vi "Query Instrument for ID and Name.vi"(0 "VISA resource name":refnum<visa-resource-name>, 11 "error in (no error)":errorcluster) -> (4 "VISA resource name out":refnum<visa-resource-name>, 6 "Logical Instrument Number":u32 max=12 step=1, 8 "Logical Instrument Name":string, 15 "error out":errorcluster)   [LabVIEW 2020, in "NH Research Regenerative Test Series.lvlib"]
doc: "Returns the <B>Logical Instrument Number</B> and <B>Logical Instrument Name</B> of the selected instrument.\n\nNOTE: The 4900 only has one logical instrument so the only valid instrument number is 1."
uses:
  NH Research Regenerative Test Series.lvlib
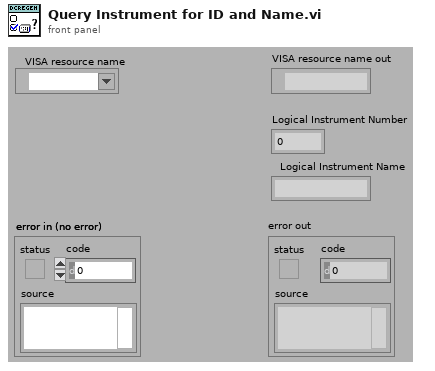
[diagram p1: front panel]
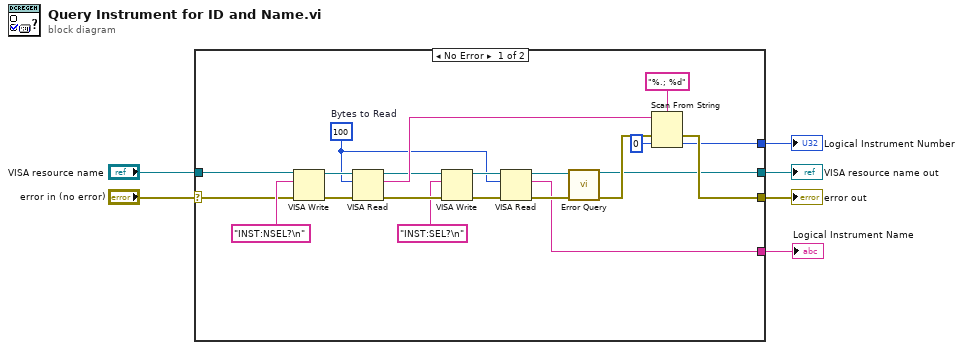
[diagram p0: block diagram]
diagram:
  n1 = case shown="No Error" "error in (no error)" {
    selector: "error in (no error)" -> [w18 w29]
    tunnel: "VISA resource name" -> [w27 w28]
    tunnel: [w20 w28] -> w5
    tunnel: [w21 w29] -> w4
    tunnel: [w7 _] -> w2
    tunnel: [w10 _] -> w1
    frame No Error {
      w9 = u32 100  # Bytes to Read
      n2 = VISA Write(VISA resource name=w27, write buffer="INST:NSEL?\n" ("Command"), error in (no error)=w18) -> (VISA resource name out=w22:refnum<visa-resource-name>, error out=w23:errorcluster)  [unwired: 1 out]
      n3 = VISA Read(VISA resource name=w22, byte count=w9, error in (no error)=w23) -> (VISA resource name out=w13:refnum<visa-resource-name>, read buffer=w26:string, error out=w15:errorcluster)  [unwired: 1 out]
      n4 = VISA Write(VISA resource name=w13, write buffer="INST:SEL?\n" ("Command"), error in (no error)=w15) -> (VISA resource name out=w16:refnum<visa-resource-name>, error out=w17:errorcluster)  [unwired: 1 out]
      n5 = VISA Read(VISA resource name=w16, byte count=w9, error in (no error)=w17) -> (VISA resource name out=w12:refnum<visa-resource-name>, read buffer=w10:string, error out=w14:errorcluster)  [unwired: 1 out]
      n6 = call "Error Query.vi"("VISA resource name"=w12, "error in (no error)"=w14) -> ("VISA resource name out"=w20:refnum<visa-resource-name>, "error out"=w24:errorcluster)  [unwired: 10 in, 2 out]
      n7 = Scan From String(format string="%.; %d", input string=w26, error in=w24, default 1=u32 0 ("default value 1")) -> (error out=w21:errorcluster, output 1=w7:u32)  [unwired: 1 in, 2 out]
    }
    frame Error {
    }
  }
  "error out" <- w4
  "VISA resource name out" <- w5
  "Logical Instrument Number" <- w2
  "Logical Instrument Name" <- w1
